vi "Sort_2D_String_array.vi"(2 "Column index to sort on":i32, 3 "arrayIn":string[][](array[string])) -> (0 "Sort Index":i32[](array[numeric]), 1 "arrayOut":string[][](array[string]))   [LabVIEW 2020]
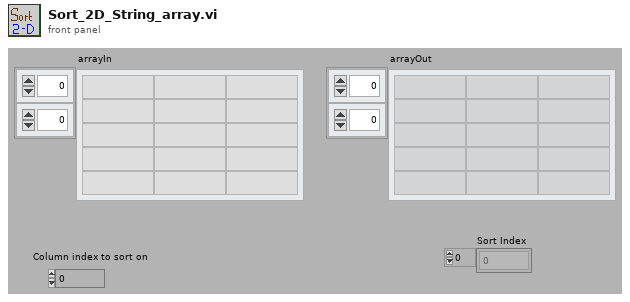
[diagram p1: front panel]
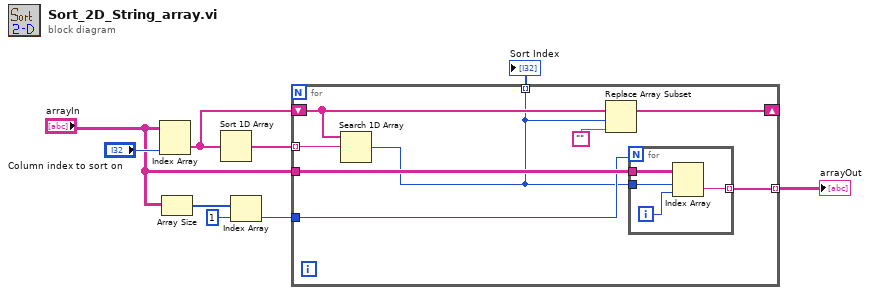
[diagram p0: block diagram]
diagram:
  n1 = Index Array(array="arrayIn", index (col)="Column index to sort on") -> (element=w4:string[])  [unwired: 1 in]
  n2 = Array Size(array="arrayIn") -> (size(s)=w7:i32[])
  n3 = Sort 1D Array(array=w4) -> (sorted array=w9:string[])
  n4 = Index Array(array=w7, index=1) -> (element=w5:i32)
  n5 = for {
    tunnel: w9 -> [w17] mode=indexing
    tunnel: "arrayIn" -> [w16]
    tunnel: [w15] -> w1 mode=indexing
    tunnel: w5 -> [w14]
    shift-right: [w12] -> _
    shift-left: w4 -> [w13]
    tunnel: [w11] -> w3 mode=indexing
    n6 = Search 1D Array(1D array=w13, element=w17) -> (index of element=w11:i32)  [unwired: 1 in]
    n7 = Replace Array Subset(array=w13, new element="", index=w11) -> (w12:string[])
    n8 = for {
      N: w14 -> [_]
      tunnel: w16 -> [w21]
      tunnel: w11 -> [w19]
      tunnel: [w18] -> w15 mode=indexing
      i -> [w20]
      n9 = Index Array(array=w21, index (row)=w19, index (col)=w20) -> (element=w18:string)
    }
  }
  "Sort Index" <- w3
  "arrayOut" <- w1
